vi "rsscope_core_global.vi"() -> ()   [LabVIEW 2018] (continued)
Options"="", "Flags"=0, "Help"="Defines for the selected field, how an index check is executed."}, {"Level"=5, "Class Only"=FALSE, "Identifier"="RSSCOPE_ATTR_USB_PD_SEARCH_INDEX_CONDITION", "Descriptive Name"="USB PD Search Index Condition", "Data Type"=0, "Command"="SEAR:TRIG:USBP:FRAM:FIEL{FieldNumber}:IOP", "Access"=2, "Range Table"="rsscope_rngUSB31Gen1IndexCondition", "Read Callback"="rsscope_FormatUSBPDPacketTypeInt32_ReadCallback.vi", "Write Callback"="rsscope_FormatUSBPDPacketTypeInt32_WriteCallback.vi", "Supported Models"="", "Instrument Options"="K63", "Flags"=0, "Help"="Sets the operator for the index in the selected field of the selected frame.\n\nAvailable Repeated Capabilities:\nFieldNumber: Field1, Field2, Field3, Field4, Field5, Field6, Field7, Field8, Field9, Field10, Field11, Field12, Field13, Field14, Field15, Field16, Field17, Field18, Field19, Field20\r\n\nRemote-control command(s):\nSEARch:TRIGger:USBPd:FRAMe:FIELd<m>:IOPerator"}, {"Level"=5, "Class Only"=FALSE, "Identifier"="RSSCOPE_ATTR_USB_PD_SEARCH_INDEX_MIN", "Descriptive Name"="USB PD Search Index Min", "Data Type"=0, "Command"="SEAR:TRIG:USBP:FRAM:FIEL{FieldNumber}:IMIN", "Access"=2, "Range Table"="", "Read Callback"="rsscope_FormatUSBPDPacketTypeInt32_ReadCallback.vi", "Write Callback"="rsscope_FormatUSBPDPacketTypeInt32_WriteCallback.vi", "Supported Models"="", "Instrument Options"="K63", "Flags"=0, "Help"="Specifies a data bit pattern, or sets the start value of a pattern range.\n\nValid Values:\nBinary pattern string consisting of 1; 0; or X (any bit).\n\nAvailable Repeated Capabilities:\nFieldNumber: Field1, Field2, Field3, Field4, Field5, Field6, Field7, Field8, Field9, Field10, Field11, Field12, Field13, Field14, Field15, Field16, Field17, Field18, Field19, Field20\r\n\nRemote-control command(s):\nSEARch:TRIGger:USBPd:FRAMe:FIELd<m>:IMIN"}, {"Level"=5, "Class Only"=FALSE, "Identifier"="RSSCOPE_ATTR_USB_PD_SEARCH_INDEX_MAX", "Descriptive Name"="USB PD Search Index Max", "Data Type"=0, "Command"="SEAR:TRIG:USBP:FRAM:FIEL{FieldNumber}:IMAX", "Access"=2, "Range Table"="", "Read Callback"="rsscope_FormatUSBPDPacketTypeInt32_ReadCallback.vi", "Write Callback"="rsscope_FormatUSBPDPacketTypeInt32_WriteCallback.vi", "Supported Models"="", "Instrument Options"="K63", "Flags"=0, "Help"="Sets the end value of a data type range for condition In Range or Out of Range. \n\nValid Values:\nBinary pattern string consisting of 1; 0; or X (any bit).\n\nAvailable Repeated Capabilities:\nFieldNumber: Field1, Field2, Field3, Field4, Field5, Field6, Field7, Field8, Field9, Field10, Field11, Field12, Field13, Field14, Field15, Field16, Field17, Field18, Field19, Field20\r\n\nRemote-control command(s):\nSEARch:TRIGger:USBPd:FRAMe:FIELd<m>:IMAX"}, {"Level"=4, "Class Only"=TRUE, "Identifier"="", "Descriptive Name"="Bit State", "Data Type"=0, "Command"="", "Access"=0, "Range Table"="", "Read Callback"="", "Write Callback"="", "Supported Models"="", "Instrument Options"="", "Flags"=0, "Help"="Defines the bit state to be checked for the selected field. Permitted bit states are 1, 0 or X (don&apos;t care)."}, {"Level"=5, "Class Only"=FALSE, "Identifier"="RSSCOPE_ATTR_USB_PD_SEARCH_BIT_STATE", "Descriptive Name"="USB PD Search Bit State", "Data Type"=0, "Command"="SEAR:TRIG:USBP:FRAM:FIEL{FieldNumber}:BIT", "Access"=2, "Range Table"="RsScope_rngBitState", "Read Callback"="rsscope_FormatUSBPDPacketTypeInt32_ReadCallback.vi", "Write Callback"="rsscope_FormatUSBPDPacketTypeInt32_WriteCallback.vi", "Supported Models"="", "Instrument Options"="K63", "Flags"=0, "Help"="Sets the bit state of a field that only consists of one bit.\n\nAvailable Repeated Capabilities:\nFieldNumber: Field1, Field2, Field3, Field4, Field5, Field6, Field7, Field8, Field9, Field10, Field11, Field12, Field13, Field14, Field15, Field16, Field17, Field18, Field19, Field20\r\n\nRemote-control command(s):\nSEARch:TRIGger:USBPd:FRAMe:FIELd<m>:BIT"}, {"Level"=4, "Class Only"=TRUE, "Identifier"="", "Descriptive Name"="Results", "Data Type"=0, "Command"="", "Access"=0, "Range Table"="", "Read Callback"="", "Write Callback"="", "Supported Models"="", "Instrument Options"="", "Flags"=0, "Help"="Returns the USB PD search results."}, {"Level"=5, "Class Only"=FALSE, "Identifier"="RSSCOPE_ATTR_SEARCH_USB_PD_FRAME_COUNT", "Descriptive Name"="Search USB PD Frame Count", "Data Type"=0, "Command"="SEAR:RES:USBP:FCO?", "Access"=0, "Range Table"="", "Read Callback"="rsscope_FormatSearchNameInt32_ReadCallback.vi", "Write Callback"="", "Supported Models"="", "Instrument Options"="K63", "Flags"=0, "Help"="Returns the number of frames in the acquisition.\n\nAvailable Repeated Capabilities:\nNone\n\nRemote-control command(s):\nSEARch:RESult:USBPd:FCOunt?"}, {"Level"=3, "Class Only"=TRUE, "Identifier"="", "Descriptive Name"="Custom Manchester NRZ", "Data Type"=0, "Command"="", "Access"=0, "Range Table"="", "Read Callback"="", "Write Callback"="", "Supported Models"="", "Instrument Options"="", "Flags"=0, "Help"="Configures Custom Manchester NRZ search"}, {"Level"=4, "Class Only"=TRUE, "Identifier"="", "Descriptive Name"="Results", "Data Type"=0, "Command"="", "Access"=0, "Range Table"="", "Read Callback"="", "Write Callback"="", "Supported Models"="", "Instrument Options"="", "Flags"=0, "Help"="Returns the search results."}, {"Level"=3, "Class Only"=TRUE, "Identifier"="", "Descriptive Name"="EbTb", "Data Type"=0, "Command"="", "Access"=0, "Range Table"="", "Read Callback"="", "Write Callback"="", "Supported Models"="", "Instrument Options"="", "Flags"=0, "Help"="The 8b/10b (Option R&S RTO-K52) coding scheme is used for high-speed serial data transmission, used by different standards, like fibre channel, PCIe, DVI and USB 3.0. Also the MIPI UniPro M-PHY interface in smartphones as well as display interfaces such as HDMI use 8b/10b encoding, as do base stations based on the Common Public Radio Interface (CPRI)."}, {"Level"=4, "Class Only"=FALSE, "Identifier"="RSSCOPE_ATTR_SEARCH_EBTB_TYPE", "Descriptive Name"="Search EbTb Type", "Data Type"=0, "Command"="SEAR:TRIG:EBTB:TYPE", "Access"=2, "Range Table"="RsScope_rngEbTbTriggerType", "Read Callback"="rsscope_FormatSearchNameInt32_ReadCallback.vi", "Write Callback"="rsscope_FormatSearchNameInt32_WriteCallback.vi", "Supported Models"="", "Instrument Options"="K52", "Flags"=0, "Help"="Selects the type of condition to be searched for. You can search for a certain symbol or enable a specific error condition.\n\nAvailable Repeated Capabilities:\nNone\n\nRemote-control command(s):\nSEARch:TRIGger:EBTB:TYPE"}, {"Level"=4, "Class Only"=FALSE, "Identifier"="RSSCOPE_ATTR_SEARCH_EBTB_DISPARITY_ERROR", "Descriptive Name"="Search EbTb Disparity Error", "Data Type"=3, "Command"="SEAR:TRIG:EBTB:DISP", "Access"=2, "Range Table"="", "Read Callback"="rsscope_FormatSearchNameBoolean_ReadCallback.vi", "Write Callback"="rsscope_FormatSearchNameBoolean_WriteCallback.vi", "Supported Models"="", "Instrument Options"="K52", "Flags"=0, "Help"="Searches for disparity errors.\n\nAvailable Repeated Capabilities:\nNone\n\nRemote-control command(s):\nSEARch:TRIGger:EBTB:DISParityerr"}, {"Level"=4, "Class Only"=FALSE, "Identifier"="RSSCOPE_ATTR_SEARCH_EBTB_GLITCHING_ERROR", "Descriptive Name"="Search EbTb Glitching Error", "Data Type"=3, "Command"="SEAR:TRIG:EBTB:GLIT", "Access"=2, "Range Table"="", "Read Callback"="rsscope_FormatSearchNameBoolean_ReadCallback.vi", "Write Callback"="rsscope_FormatSearchNameBoolean_WriteCallback.vi", "Supported Models"="", "Instrument Options"="K52", "Flags"=0, "Help"="Searches for glitching errors.\n\nAvailable Repeated Capabilities:\nNone\n\nRemote-control command(s):\nSEARch:TRIGger:EBTB:GLITcherror"}, {"Level"=4, "Class Only"=FALSE, "Identifier"="RSSCOPE_ATTR_SEARCH_EBTB_UNKNOWN_SYMBOL_ERROR", "Descriptive Name"="Search EbTb Unknown Symbol Error", "Data Type"=3, "Command"="SEAR:TRIG:EBTB:UNK", "Access"=2, "Range Table"="", "Read Callback"="rsscope_FormatSearchNameBoolean_ReadCallback.vi", "Write Callback"="rsscope_FormatSearchNameBoolean_WriteCallback.vi", "Supported Models"="", "Instrument Options"="K52", "Flags"=0, "Help"="Defines, whether a search for any unknown symbol error shall be activated or not.\n\nAvailable Repeated Capabilities:\nNone\n\nRemote-control command(s):\nSEARch:TRIGger:EBTB:UNK"}, {"Level"=4, "Class Only"=FALSE, "Identifier"="RSSCOPE_ATTR_SEARCH_EBTB_SEARCH_TYPE", "Descriptive Name"="Search EbTb Search Type", "Data Type"=0, "Command"="SEAR:TRIG:EBTB:STYP", "Access"=2, "Range Table"="RsScope_rngEbTbSearchType", "Read Callback"="rsscope_FormatSearchNameInt32_ReadCallback.vi", "Write Callback"="rsscope_FormatSearchNameInt32_WriteCallback.vi", "Supported Models"="", "Instrument Options"="K52", "Flags"=0, "Help"="Selects the search type.\n\nAvailable Repeated Capabilities:\nNone\n\nRemote-control command(s):\nSEARch:TRIGger:EBTB:STYPe"}, {"Level"=4, "Class Only"=FALSE, "Identifier"="RSSCOPE_ATTR_SEARCH_EBTB_SYMBOL_TYPE", "Descriptive Name"="Search EbTb Symbol Type", "Data Type"=0, "Command"="SEAR:TRIG:EBTB:SSTY", "Access"=2, "Range Table"="RsScope_rngEbTbSymbolType", "Read Callback"="rsscope_FormatSearchNameInt32_ReadCallback.vi", "Write Callback"="rsscope_FormatSearchNameInt32_WriteCallback.vi", "Supported Models"="", "Instrument Options"="K52", "Flags"=0, "Help"="Selects the symbol type to be searched for. You can select a single symbol or an expression (defined series of symbols).\n\nAvailable Repeated Capabilities:\nNone\n\nRemote-control command(s):\nSEARch:TRIGger:EBTB:SSTYpe"}, {"Level"=4, "Class Only"=FALSE, "Identifier"="RSSCOPE_ATTR_SEARCH_EBTB_SYMBOL_FORMAT", "Descriptive Name"="Search EbTb Symbol Format", "Data Type"=0, "Command"="SEAR:TRIG:EBTB:SYMF", "Access"=2, "Range Table"="RsScope_rngEbTbFormat", "Read Callback"="rsscope_FormatSearchNameInt32_ReadCallback.vi", "Write Callback"="rsscope_FormatSearchNameInt32_WriteCallback.vi", "Supported Models"="", "Instrument Options"="K52", "Flags"=0, "Help"="Selects the format of the symbol to be searched for, if &apos;Symbol Type&apos; > &apos;Symbol&apos;.\n\nAvailable Repeated Capabilities:\nNone\n\nRemote-control command(s):\nSEARch:TRIGger:EBTB:SYMFormat"}, {"Level"=4, "Class Only"=FALSE, "Identifier"="RSSCOPE_ATTR_SEARCH_EBTB_KD_CODE_SYMBOL", "Descriptive Name"="Search EbTb KD Code Symbol", "Data Type"=0, "Command"="SEAR:TRIG:EBTB:SYMT", "Access"=2, "Range Table"="RsScope_rngEbTbKDCode", "Read Callback"="rsscope_FormatSearchNameInt32_ReadCallback.vi", "Write Callback"="rsscope_FormatSearchNameInt32_WriteCallback.vi", "Supported Models"="", "Instrument Options"="K52", "Flags"=0, "Help"="Selects the data character (Dx.y) or control character to be searched for. You can specify the value of the data character to be searched for with &apos;Dx Value&apos; and &apos;Dy Value&apos;.\n\nAvailable Repeated Capabilities:\nNone\n\nRemote-control command(s):\nSEARch:TRIGger:EBTB:SYMType"}, {"Level"=4, "Class Only"=FALSE, "Identifier"="RSSCOPE_ATTR_SEARCH_EBTB_DX", "Descriptive Name"="Search EbTb Dx", "Data Type"=0, "Command"="SEAR:TRIG:EBTB:DX", "Access"=2, "Range Table"="RsScope_rngEbTbDx", "Read Callback"="rsscope_FormatSearchNameInt32_ReadCallback.vi", "Write Callback"="rsscope_FormatSearchNameInt32_WriteCallback.vi", "Supported Models"="", "Instrument Options"="K52", "Flags"=0, "Help"="Sets the x value of the data character Dx.y to be searched for, if &apos;K/D Codes Symbol&apos; > &apos;Dx.y&apos;.\n\nAvailable Repeated Capabilities:\nNone\n\nRemote-control command(s):\nSEARch:TRIGger:EBTB:DX"}, {"Level"=4, "Class Only"=FALSE, "Identifier"="RSSCOPE_ATTR_SEARCH_EBTB_DY", "Descriptive Name"="Search EbTb Dy", "Data Type"=0, "Command"="SEAR:TRIG:EBTB:DY", "Access"=2, "Range Table"="RsScope_rngEbTbDy", "Read Callback"="rsscope_FormatSearchNameInt32_ReadCallback.vi", "Write Callback"="rsscope_FormatSearchNameInt32_WriteCallback.vi", "Supported Models"="", "Instrument Options"="K52", "Flags"=0, "Help"="Sets the y value of the data character Dx.y to be searched for, if &apos;K/D Codes Symbol&apos; > &apos;Dx.y&apos;.\n\nAvailable Repeated Capabilities:\nNone\n\nRemote-control command(s):\nSEARch:TRIGger:EBTB:DY"}, {"Level"=4, "Class Only"=FALSE, "Identifier"="RSSCOPE_ATTR_SEARCH_EBTB_EIGHT_BIT_PATTERN", "Descriptive Name"="Search EBTB Eight Bit Pattern", "Data Type"=2, "Command"="SEAR:TRIG:EBTB:EBPA", "Access"=2, "Range Table"="", "Read Callback"="rsscope_FormatSearchNameString_ReadCallback.vi", "Write Callback"="rsscope_FormatSearchNameString_WriteCallback.vi", "Supported Models"="", "Instrument Options"="K52", "Flags"=0, "Help"="Sets the 8-bit pattern to be searched for, if &apos;Format&apos; > &apos;8-bit&apos;.\n \nNote(s):\n(1) Valid values 1; 0; or X (any bit), use of X is restricted to the conditions &apos;Equal&apos; and &apos;Not equal&apos;.\n\nAvailable Repeated Capabilities:\nNone\n\nRemote-control command(s):\nSEARch:TRIGger:EBTB:EBPA"}, {"Level"=4, "Class Only"=FALSE, "Identifier"="RSSCOPE_ATTR_SEARCH_EBTB_TEN_BIT_PATTERN", "Descriptive Name"="Search EBTB Ten Bit Pattern", "Data Type"=2, "Command"="SEAR:TRIG:EBTB:TBPA", "Access"=2, "Range Table"="", "Read Callback"="rsscope_FormatSearchNameString_ReadCallback.vi", "Write Callback"="rsscope_FormatSearchNameString_WriteCallback.vi", "Supported Models"="", "Instrument Options"="K52", "Flags"=0, "Help"="Sets the 10-bit pattern to be searched for, if &apos;Format&apos; > &apos;10-bit&apos;.\n \nNote(s):\n(1) Valid values 1; 0; or X (any bit), use of X is restricted to the conditions &apos;Equal&apos; and &apos;Not equal&apos;.\n\nAvailable Repeated Capabilities:\nNone\n\nRemote-control command(s):\nSEARch:TRIGger:EBTB:TBPA"}, {"Level"=4, "Class Only"=FALSE, "Identifier"="RSSCOPE_ATTR_SEARCH_EBTB_EXPRESSION", "Descriptive Name"="Search EBTB Expression", "Data Type"=2, "Command"="SEAR:TRIG:EBTB:SYME", "Access"=2, "Range Table"="", "Read Callback"="rsscope_FormatSearchNameString_ReadCallback.vi", "Write Callback"="rsscope_FormatSearchNameString_WriteCallback.vi", "Supported Models"="", "Instrument Options"="K52", "Flags"=0, "Help"="Defines the expression to be searched for, if &apos;Symbol Type&apos; > &apos;Expression&apos;.\n\nAvailable Repeated Capabilities:\nNone\n\nRemote-control command(s):\nSEARch:TRIGger:EBTB:SYME"}, {"Level"=4, "Class Only"=TRUE, "Identifier"="", "Descriptive Name"="Results", "Data Type"=0, "Command"="", "Access"=0, "Range Table"="", "Read Callback"="", "Write Callback"="", "Supported Models"="", "Instrument Options"="", "Flags"=0, "Help"="Returns the search results."}, {"Level"=5, "Class Only"=FALSE, "Identifier"="RSSCOPE_ATTR_SEARCH_EBTB_SYMBOL_COUNT", "Descriptive Name"="Search EbTb Symbol Count", "Data Type"=0, "Command"="SEAR:RES:EBTB:SCO?", "Access"=0, "Range Table"="", "Read Callback"="rsscope_FormatSearchNameInt32_ReadCallback.vi", "Write Callback"="", "Supported Models"="", "Instrument Options"="K52", "Flags"=0, "Help"="Returns the symbol count for the selected serial bus, i.e. the number of symbols in the present acquisition.\n\nAvailable Repeated Capabilities:\nNone\n\nRemote-control command(s):\nSEARch:RESult:EBTB:SCOunt?"}, {"Level"=3, "Class Only"=TRUE, "Identifier"="", "Descriptive Name"="SENT", "Data Type"=0, "Command"="", "Access"=0, "Range Table"="", "Read Callback"="", "Write Callback"="", "Supported Models"="", "Instrument Options"="", "Flags"=0, "Help"="SENT (Single Ended Nibble Transmission, R&S RTO-K10 option) is a serial transmission interface protocol originally specified for the communication of sensors and control units in automotive electronics."}, {"Level"=4, "Class Only"=FALSE, "Identifier"="RSSCOPE_ATTR_SEARCH_SENT_CALIBRATION_ENABLED", "Descriptive Name"="Search SENT Calibration Enabled", "Data Type"=3, "Command"="SEAR:TRIG:SENT:CAL", "Access"=2, "Range Table"="", "Read Callback"="rsscope_FormatSearchNameBoolean_ReadCallback.vi", "Write Callback"="rsscope_FormatSearchNameBoolean_WriteCallback.vi", "Supported Models"="", "Instrument Options"="K10", "Flags"=0, "Help"="Enables the search for the Calibration/Synchronization pulse.\n\nAvailable Repeated Capabilities:\nNone\n\nRemote-control command(s):\nSEARch:TRIGger:SENT:CALibration"}, {"Level"=4, "Class Only"=TRUE, "Identifier"="", "Descriptive Name"="Transmission Sequence", "Data Type"=0, "Command"="", "Access"=0, "Range Table"="", "Read Callback"="", "Write Callback"="", "Supported Models"="", "Instrument Options"="", "Flags"=0, "Help"="Configures the trigger conditions for trigger type transmission sequence."}, {"Level"=5, "Class Only"=FALSE, "Identifier"="RSSCOPE_ATTR_SEARCH_SENT_TRANSMISSION_SEQUENCE_ENABLED", "Descriptive Name"="Search SENT Transmission Sequence Enabled", "Data Type"=3, "Command"="SEAR:TRIG:SENT:TRAN", "Access"=2, "Range Table"="", "Read Callback"="rsscope_FormatSearchNameBoolean_ReadCallback.vi", "Write Callback"="rsscope_FormatSearchNameBoolean_WriteCallback.vi", "Supported Models"="", "Instrument Options"="K10", "Flags"=0, "Help"="Enables the search for a transmission sequence.\n\nAvailable Repeated Capabilities:\nNone\n\nRemote-control command(s):\nSEARch:TRIGger:SENT:TRANsmission"}, {"Level"=5, "Class Only"=FALSE, "Identifier"="RSSCOPE_ATTR_SEARCH_SENT_TRANSMISSION_SEQUENCE_TYPE", "Descriptive Name"="Search SENT Transmission Sequence Type", "Data Type"=0, "Command"="SEAR:TRIG:SENT:TTYP", "Access"=2, "Range Table"="RsScope_rngSENTTriggerTSType", "Read Callback"="rsscope_FormatSearchNameInt32_ReadCallback.vi", "Write Callback"="rsscope_FormatSearchNameInt32_WriteCallback.vi", "Supported Models"="", "Instrument Options"="K10", "Flags"=0, "Help"="Selects the SENT transmission sequence to be searched for.\n\nAvailable Repeated Capabilities:\nNone\n\nRemote-control command(s):\nSEARch:TRIGger:SENT:TTYPe"}, {"Level"=5, "Class Only"=FALSE, "Identifier"="RSSCOPE_ATTR_SEARCH_SENT_TRANSMISSION_SEQUENCE_STATUS", "Descriptive Name"="Search SENT Transmission Sequence Status", "Data Type"=2, "Command"="SEAR:TRIG:SENT:STAT", "Access"=2, "Range Table"="", "Read Callback"="rsscope_FormatSearchNameString_ReadCallback.vi", "Write Callback"="rsscope_FormatSearchNameString_WriteCallback.vi", "Supported Models"="", "Instrument Options"="K10", "Flags"=0, "Help"="Sets the status nibble data, numeric or string pattern. The string parameter accepts the bit value X (don&apos;t care).\n\nAvailable Repeated Capabilities:\nNone\n\nRemote-control command(s):\nSEARch:TRIGger:SENT:STATus"}, {"Level"=5, "Class Only"=FALSE, "Identifier"="RSSCOPE_ATTR_SEARCH_SENT_TRANSMISSION_SEQUENCE_CONDITION", "Descriptive Name"="Search SENT Transmission Sequence Condition", "Data Type"=0, "Command"="SEAR:TRIG:SENT:TDCN", "Access"=2, "Range Table"="rsscope_rngProtocolTriggerCondition", "Read Callback"="rsscope_FormatSearchNameInt32_ReadCallback.vi", "Write Callback"="rsscope_FormatSearchNameInt32_WriteCallback.vi", "Supported Models"="", "Instrument Options"="K10", "Flags"=0, "Help"="Sets the operator to set a specific data pattern or a data pattern range.\n\nAvailable Repeated Capabilities:\nNone\n\nRemote-control command(s):\nSEARch:TRIGger:SENT:TDCN"}, {"Level"=5, "Class Only"=FALSE, "Identifier"="RSSCOPE_ATTR_SEARCH_SENT_TRANSMISSION_SEQUENCE_DATA_MIN", "Descriptive Name"="Search SENT Transmission Sequence Data Min", "Data Type"=2, "Command"="SEAR:TRIG:SENT:TDMN", "Access"=2, "Range Table"="", "Read Callback"="rsscope_FormatSearchNameString_ReadCallback.vi", "Write Callback"="rsscope_FormatSearchNameString_WriteCallback.vi", "Supported Models"="", "Instrument Options"="K10", "Flags"=0, "Help"="Specifies a data pattern, or sets the start value of a data pattern range. The string parameter accepts the bit value X (don&apos;t care).\n\nAvailable Repeated Capabilities:\nNone\n\nRemote-control command(s):\nSEARch:TRIGger:SENT:TDMN"}, {"Level"=5, "Class Only"=FALSE, "Identifier"="RSSCOPE_ATTR_SEARCH_SENT_TRANSMISSION_SEQUENCE_DATA_MAX", "Descriptive Name"="Search SENT Transmission Sequence Data Max", "Data Type"=2, "Command"="SEAR:TRIG:SENT:TDMX", "Access"=2, "Range Table"="", "Read Callback"="rsscope_FormatSearchNameString_ReadCallback.vi", "Write Callback"="rsscope_FormatSearchNameString_WriteCallback.vi", "Supported Models"="", "Instrument Options"="K10", "Flags"=0, "Help"="Sets the end value of an identifier range for condition In Range or Out of Range. The string parameter accepts the bit value X (don&apos;t care).\n\nAvailable Repeated Capabilities:\nNone\n\nRemote-control command(s):\nSEARch:TRIGger:SENT:TDMX"}, {"Level"=4, "Class Only"=TRUE, "Identifier"="", "Descriptive Name"="Serial Message", "Data Type"=0, "Command"="", "Access"=0, "Range Table"="", "Read Callback"="", "Write Callback"="", "Supported Models"="", "Instrument Options"="", "Flags"=0, "Help"="Configures the trigger conditions for a serial message."}, {"Level"=5, "Class Only"=FALSE, "Identifier"="RSSCOPE_ATTR_SEARCH_SENT_SERIAL_MESSAGE_ENABLED", "Descriptive Name"="Search SENT Serial Message Enabled", "Data Type"=3, "Command"="SEAR:TRIG:SENT:SMSG", "Access"=2, "Range Table"="", "Read Callback"="rsscope_FormatSearchNameBoolean_ReadCallback.vi", "Write Callback"="rsscope_FormatSearchNameBoolean_WriteCallback.vi", "Supported Models"="", "Instrument Options"="K10", "Flags"=0, "Help"="Enables the search in a serial message.\n\nAvailable Repeated Capabilities:\nNone\n\nRemote-control command(s):\nSEARch:TRIGger:SENT:SMSG"}, {"Level"=5, "Class Only"=FALSE, "Identifier"="RSSCOPE_ATTR_SEARCH_SENT_SERIAL_MESSAGE_TYPE", "Descriptive Name"="Search SENT Serial Message Type", "Data Type"=0, "Command"="SEAR:TRIG:SENT:STYP", "Access"=2, "Range Table"="RsScope_rngSENTTriggerSMType", "Read Callback"="rsscope_FormatSearchNameInt32_ReadCallback.vi", "Write Callback"="rsscope_FormatSearchNameInt32_WriteCallback.vi", "Supported Models"="", "Instrument Options"="K10", "Flags"=0, "Help"="Selects the serial message sequence to be searched for.\n\nAvailable Repeated Capabilities:\nNone\n\nRemote-control command(s):\nSEARch:TRIGger:SENT:STYPe"}, {"Level"=5, "Class Only"=FALSE, "Identifier"="RSSCOPE_ATTR_SEARCH_SENT_SERIAL_MESSAGE_ID_TYPE", "Descriptive Name"="Search SENT Serial Message ID Type", "Data Type"=0, "Command"="SEAR:TRIG:SENT:SIDT", "Access"=2, "Range Table"="RsScope_rngSENTIDType", "Read Callback"="rsscope_FormatSearchNameInt32_ReadCallback.vi", "Write Callback"="rsscope_FormatSearchNameInt32_WriteCallback.vi", "Supported Models"="", "Instrument Options"="K10", "Flags"=0, "Help"="Sets the message ID format (4 bit or 8 bit) of the enhanced serial message.\n\nAvailable Repeated Capabilities:\nNone\n\nRemote-control command(s):\nSEARch:TRIGger:SENT:SIDType"}, {"Level"=5, "Class Only"=FALSE, "Identifier"="RSSCOPE_ATTR_SEARCH_SENT_SERIAL_MESSAGE_ID_CONDITION", "Descriptive Name"="Search SENT Serial Message ID Condition", "Data Type"=0, "Command"="SEAR:TRIG:SENT:SICN", "Access"=2, "Range Table"="rsscope_rngProtocolTriggerCondition", "Read Callback"="rsscope_FormatSearchNameInt32_ReadCallback.vi", "Write Callback"="rsscope_FormatSearchNameInt32_WriteCallback.vi", "Supported Models"="", "Instrument Options"="K10", "Flags"=0, "Help"="Sets the operator to set a specific data pattern or a data pattern range.\n\nAvailable Repeated Capabilities:\nNone\n\nRemote-control command(s):\nSEARch:TRIGger:SENT:SICN"}, {"Level"=5, "Class Only"=FALSE, "Identifier"="RSSCOPE_ATTR_SEARCH_SENT_SERIAL_MESSAGE_ID_MIN", "Descriptive Name"="Search SENT Serial Message ID Min", "Data Type"=2, "Command"="SEAR:TRIG:SENT:SIMN", "Access"=2, "Range Table"="", "Read Callback"="rsscope_FormatSearchNameString_ReadCallback.vi", "Write Callback"="rsscope_FormatSearchNameString_WriteCallback.vi", "Supported Models"="", "Instrument Options"="K10", "Flags"=0, "Help"="Specifies a message identifier pattern, or sets the start value of an identifier range. The string parameter accepts the bit value X (don&apos;t care).\n\nAvailable Repeated Capabilities:\nNone\n\nRemote-control command(s):\nSEARch:TRIGger:SENT:SIMN"}, {"Level"=5, "Class Only"=FALSE, "Identifier"="RSSCOPE_ATTR_SEARCH_SENT_SERIAL_MESSAGE_ID_MAX", "Descriptive Name"="Search SENT Serial Message ID Max", "Data Type"=2, "Command"="SEAR:TRIG:SENT:SIMX", "Access"=2, "Range Table"="", "Read Callback"="rsscope_FormatSearchNameString_ReadCallback.vi", "Write Callback"="rsscope_FormatSearchNameString_WriteCallback.vi", "Supported Models"="", "Instrument Options"="K10", "Flags"=0, "Help"="Sets the end value of an identifier range for condition In Range or Out of Range. The string parameter accepts the bit value X (don&apos;t care).\n\nAvailable Repeated Capabilities:\nNone\n\nRemote-control command(s):\nSEARch:TRIGger:SENT:SIMX"}, {"Level"=5, "Class Only"=FALSE, "Identifier"="RSSCOPE_ATTR_SEARCH_SENT_SERIAL_MESSAGE_DATA_CONDITION", "Descriptive Name"="Search SENT Serial Message Data Condition", "Data Type"=0, "Command"="SEAR:TRIG:SENT:SDCN", "Access"=2, "Range Table"="rsscope_rngProtocolTriggerCondition", "Read Callback"="rsscope_FormatSearchNameInt32_ReadCallback.vi", "Write Callback"="rsscope_FormatSearchNameInt32_WriteCallback.vi", "Supported Models"="", "Instrument Options"="K10", "Flags"=0, "Help"="Sets the operator to define a specific data pattern or a data pattern range.\n\nAvailable Repeated Capabilities:\nNone\n\nRemote-control command(s):\nSEARch:TRIGger:SENT:SDCN"}, {"Level"=5, "Class Only"=FALSE, "Identifier"="RSSCOPE_ATTR_SEARCH_SENT_SERIAL_MESSAGE_DATA_MIN", "Descriptive Name"="Search SENT Serial Message Data Min", "Data Type"=2, "Command"="SEAR:TRIG:SENT:SDMN", "Access"=2, "Range Table"="", "Read Callback"="rsscope_FormatSearchNameString_ReadCallback.vi", "Write Callback"="rsscope_FormatSearchNameString_WriteCallback.vi", "Supported Models"="", "Instrument Options"="K10", "Flags"=0, "Help"="Specifies a data pattern, or sets the start value of a data pattern range. The string parameter accepts the bit value X (don&apos;t care).\n\nAvailable Repeated Capabilities:\nNone\n\nRemote-control command(s):\nSEARch:TRIGger:SENT:SDMN"}, {"Level"=5, "Class Only"=FALSE, "Identifier"="RSSCOPE_ATTR_SEARCH_SENT_SERIAL_MESSAGE_DATA_MAX", "Descriptive Name"="Search SENT Serial Message Data Max", "Data Type"=2, "Command"="SEAR:TRIG:SENT:SDMX", "Access"=2, "Range Table"="", "Read Callback"="rsscope_FormatSearchNameString_ReadCallback.vi", "Write Callback"="rsscope_FormatSearchNameString_WriteCallback.vi", "Supported Models"="", "Instrument Options"="K10", "Flags"=0, "Help"="Sets the end value of an identifier range for condition In Range or Out of Range. The string parameter accepts the bit value X (don&apos;t care).\n\nAvailable Repeated Capabilities:\nNone\n\nRemote-control command(s):\nSEARch:TRIGger:SENT:SDMX"}, {"Level"=4, "Class Only"=TRUE, "Identifier"="", "Descriptive Name"="Error Conditions", "Data Type"=0, "Command"="", "Access"=0, "Range Table"="", "Read Callback"="", "Write Callback"="", "Supported Models"="", "Instrument Options"="", "Flags"=0, "Help"="This class configures conditions for Error trigger."}, {"Level"=5, "Class Only"=FALSE, "Identifier"="RSSCOPE_ATTR_SEARCH_SENT_ERROR_ENABLED", "Descriptive Name"="Search SENT Error Enabled", "Data Type"=3, "Command"="SEAR:TRIG:SENT:ERR", "Access"=2, "Range Table"="", "Read Callback"="rsscope_FormatSearchNameBoolean_ReadCallback.vi", "Write Callback"="rsscope_FormatSearchNameBoolean_WriteCallback.vi", "Supported Models"="", "Instrument Options"="K10", "Flags"=0, "Help"="Enables the search for a specified error.\n\nAvailable Repeated Capabilities:\nNone\n\nRemote-control command(s):\nSEARch:TRIGger:SENT:ERRor"}, {"Level"=5, "Class Only"=FALSE, "Identifier"="RSSCOPE_ATTR_SEARCH_SENT_FORM_ERROR", "Descriptive Name"="Search SENT Form Error", "Data Type"=3, "Command"="SEAR:TRIG:SENT:FORM", "Access"=2, "Range Table"="", "Read Callback"="rsscope_FormatSearchNameBoolean_ReadCallback.vi", "Write Callback"="rsscope_FormatSearchNameBoolean_WriteCallback.vi", "Supported Models"="", "Instrument Options"="K10", "Flags"=0, "Help"="Enables the search for format errors in serial messages.\n\nAvailable Repeated Capabilities:\nNone\n\nRemote-control command(s):\nSEARch:TRIGger:SENT:FORMerror"}, {"Level"=5, "Class Only"=FALSE, "Identifier"="RSSCOPE_ATTR_SEARCH_SENT_CALIBRATION_PULSE_ERROR", "Descriptive Name"="Search SENT Calibration Pulse Error", "Data Type"=3, "Command"="SEAR:TRIG:SENT:PULS", "Access"=2, "Range Table"="", "Read Callback"="rsscope_FormatSearchNameBoolean_ReadCallback.vi", "Write Callback"="rsscope_FormatSearchNameBoolean_WriteCallback.vi", "Supported Models"="", "Instrument Options"="K10", "Flags"=0, "Help"="Enables the search for pulse errors.\n\nAvailable Repeated Capabilities:\nNone\n\nRemote-control command(s):\nSEARch:TRIGger:SENT:PULSeerror"}, {"Level"=5, "Class Only"=FALSE, "Identifier"="RSSCOPE_ATTR_SEARCH_SENT_PULSE_PERIOD_ERROR", "Descriptive Name"="Search SENT Pulse Period Error", "Data Type"=3, "Command"="SEAR:TRIG:SENT:PPER", "Access"=2, "Range Table"="", "Read Callback"="rsscope_FormatSearchNameBoolean_ReadCallback.vi", "Write Callback"="rsscope_FormatSearchNameBoolean_WriteCallback.vi", "Supported Models"="", "Instrument Options"="K10", "Flags"=0, "Help"="Enables the search for pulse period errors.\n\nAvailable Repeated Capabilities:\nNone\n\nRemote-control command(s):\nSEARch:TRIGger:SENT:PPERioderror"}, {"Level"=5, "Class Only"=FALSE, "Identifier"="RSSCOPE_ATTR_SEARCH_SENT_CRC_ERROR", "Descriptive Name"="Search SENT CRC Error", "Data Type"=3, "Command"="SEAR:TRIG:SENT:CRC", "Access"=2, "Range Table"="", "Read Callback"="rsscope_FormatSearchNameBoolean_ReadCallback.vi", "Write Callback"="rsscope_FormatSearchNameBoolean_WriteCallback.vi", "Supported Models"="", "Instrument Options"="K10", "Flags"=0, "Help"="Enables the search for errors in the Cyclic Redundancy Check.\n\nAvailable Repeated Capabilities:\nNone\n\nRemote-control command(s):\nSEARch:TRIGger:SENT:CRCerror"}, {"Level"=5, "Class Only"=FALSE, "Identifier"="RSSCOPE_ATTR_SEARCH_SENT_IRREGULAR_FRAME_LENGTH_ERROR", "Descriptive Name"="Search SENT Irregular Frame Length Error", "Data Type"=3, "Command"="SEAR:TRIG:SENT:IRFL", "Access"=2, "Range Table"="", "Read Callback"="rsscope_FormatSearchNameBoolean_ReadCallback.vi", "Write Callback"="rsscope_FormatSearchNameBoolean_WriteCallback.vi", "Supported Models"="", "Instrument Options"="K10", "Flags"=0, "Help"="Enables the search for irregular frame length errors.\n\nAvailable Repeated Capabilities:\nNone\n\nRemote-control command(s):\nSEARch:TRIGger:SENT:IRFLength"}, {"Level"=4, "Class Only"=TRUE, "Identifier"="", "Descriptive Name"="Results", "Data Type"=0, "Command"="", "Access"=0, "Range Table"="", "Read Callback"="", "Write Callback"="", "Supported Models"="", "Instrument Options"="", "Flags"=0, "Help"="Returns the search results."}, {"Level"=5, "Class Only"=FALSE, "Identifier"="RSSCOPE_ATTR_SEARCH_SENT_FRAME_COUNT", "Descriptive Name"="Search SENT Frame Count", "Data Type"=0, "Command"="SEAR:RES:SENT:FCO?", "Access"=0, "Range Table"="", "Read Callback"="rsscope_FormatSearchNameInt32_ReadCallback.vi", "Write Callback"="", "Supported Models"="", "Instrument Options"="K10", "Flags"=0, "Help"="Returns the number of decoded frames of the acquisition.\n\nAvailable Repeated Capabilities:\nNone\n\nRemote-control command(s):\nSEARch:RESult:SENT:FCOunt?"}, {"Level"=3, "Class Only"=TRUE, "Identifier"="", "Descriptive Name"="D-PHY", "Data Type"=0, "Command"="", "Access"=0, "Range Table"="", "Read Callback"="", "Write Callback"="", "Supported Models"="", "Instrument Options"="", "Flags"=0, "Help"="In this class all search settings can be configured."}, {"Level"=4, "Class Only"=FALSE, "Identifier"="RSSCOPE_ATTR_DPHY_SEARCH_TYPE", "Descriptive Name"="DPHY Search Type", "Data Type"=0, "Command"="SEAR:TRIG:DPHY:TYPE", "Access"=2, "Range Table"="RsScope_rngDPHYTriggerType", "Read Callback"="rsscope_FormatSearchNameInt32_ReadCallback.vi", "Write Callback"="rsscope_FormatSearchNameInt32_WriteCallback.vi", "Supported Models"="", "Instrument Options"="K42", "Flags"=0, "Help"="Sets the type of frame to be searched for.\n\nAvailable Repeated Capabilities:\nNone\n\nRemote-control command(s):\nSEARch:TRIGger:DPHY:TYPE"}, {"Level"=4, "Class Only"=FALSE, "Identifier"="RSSCOPE_ATTR_DPHY_SEARCH_VIRTUAL_CHANNEL", "Descriptive Name"="DPHY Search Virtual Channel", "Data Type"=2, "Command"="SEAR:TRIG:DPHY:HSVC", "Access"=2, "Range Table"="", "Read Callback"="rsscope_FormatSearchNameString_ReadCallback.vi", "Write Callback"="rsscope_FormatSearchNameString_WriteCallback.vi", "Supported Models"="", "Instrument Options"="K42", "Flags"=0, "Help"="Sets the virtual channel to be searched for.\n\nAvailable Repeated Capabilities:\nNone\n\nRemote-control command(s):\nSEARch:TRIGger:DPHY:HSVC"}, {"Level"=4, "Class Only"=TRUE, "Identifier"="", "Descriptive Name"="Data Type", "Data Type"=0, "Command"="", "Access"=0, "Range Table"="", "Read Callback"="", "Write Callback"="", "Supported Models"="", "Instrument Options"="", "Flags"=0, "Help"="Sets the specified data type to be searched for. The data type setup consists of the condition and one or two data patterns."}, {"Level"=5, "Class Only"=FALSE, "Identifier"="RSSCOPE_ATTR_DPHY_SEARCH_DATA_TYPE_CONDITION", "Descriptive Name"="DPHY Search Data Type Condition", "Data Type"=0, "Command"="SEAR:TRIG:DPHY:DTYP:COND", "Access"=2, "Range Table"="rsscope_rngProtocolTriggerCondition", "Read Callback"="rsscope_FormatSearchNameInt32_ReadCallback.vi", "Write Callback"="rsscope_FormatSearchNameInt32_WriteCallback.vi", "Supported Models"="", "Instrument Options"="K42", "Flags"=0, "Help"="Set the condition for the data type. You can define an exact value or a value range.\n\nAvailable Repeated Capabilities:\nNone\n\nRemote-control command(s):\nSEARch:TRIGger:DPHY:DTYPe:CONDition"}, {"Level"=5, "Class Only"=FALSE, "Identifier"="RSSCOPE_ATTR_DPHY_SEARCH_DATA_TYPE_MIN", "Descriptive Name"="DPHY Search Data Type Min", "Data Type"=2, "Command"="SEAR:TRIG:DPHY:DTYP:MIN", "Access"=2, "Range Table"="", "Read Callback"="", "Write Callback"="", "Supported Models"="", "Instrument Options"="K42", "Flags"=0, "Help"="Specifies a data type pattern, or sets the start value of a pattern range.\n\nValid Values:\nBinary pattern string consisting of 1; 0; or X (any bit).\n\nAvailable Repeated Capabilities:\nNone\n\nRemote-control command(s):\nSEARch:TRIGger:DPHY:DTYPe:MIN"}, {"Level"=5, "Class Only"=FALSE, "Identifier"="RSSCOPE_ATTR_DPHY_SEARCH_DATA_TYPE_MAX", "Descriptive Name"="DPHY Search Data Type Max", "Data Type"=2, "Command"="SEAR:TRIG:DPHY:DTYP:MAX", "Access"=2, "Range Table"="", "Read Callback"="rsscope_FormatSearchNameString_ReadCallback.vi", "Write Callback"="rsscope_FormatSearchNameString_WriteCallback.vi", "Supported Models"="", "Instrument Options"="K42", "Flags"=0, "Help"="Sets the end value of a data type range for condition In Range or Out of Range. \n\nValid Values:\nBinary pattern string consisting of 1; 0; or X (any bit).\n\nAvailable Repeated Capabilities:\nNone\n\nRemote-control command(s):\nSEARch:TRIGger:DPHY:DTYPe:MAX"}, {"Level"=4, "Class Only"=TRUE, "Identifier"="", "Descriptive Name"="Word Count", "Data Type"=0, "Command"="", "Access"=0, "Range Table"="", "Read Callback"="", "Write Callback"="", "Supported Models"="", "Instrument Options"="", "Flags"=0, "Help"="Sets the specified data type to be searched for. The word count setup consists of the condition and one or two data patterns."}, {"Level"=5, "Class Only"=FALSE, "Identifier"="RSSCOPE_ATTR_DPHY_SEARCH_WORD_COUNT_CONDITION", "Descriptive Name"="DPHY Search Word Count Condition", "Data Type"=0, "Command"="SEAR:TRIG:DPHY:WCO:COND", "Access"=2, "Range Table"="rsscope_rngProtocolTriggerCondition", "Read Callback"="rsscope_FormatSearchNameInt32_ReadCallback.vi", "Write Callback"="rsscope_FormatSearchNameInt32_WriteCallback.vi", "Supported Models"="", "Instrument Options"="K42", "Flags"=0, "Help"="Set the condition for the word count. You can define an exact value or a value range.\n\nAvailable Repeated Capabilities:\nNone\n\nRemote-control command(s):\nSEARch:TRIGger:DPHY:WCOunt:CONDition"}, {"Level"=5, "Class Only"=FALSE, "Identifier"="RSSCOPE_ATTR_DPHY_SEARCH_WORD_COUNT_MIN", "Descriptive Name"="DPHY Search Word Count Min", "Data Type"=2, "Command"="SEAR:TRIG:DPHY:WCO:MIN", "Access"=2, "Range Table"="", "Read Callback"="rsscope_FormatSearchNameString_ReadCallback.vi", "Write Callback"="rsscope_FormatSearchNameString_WriteCallback.vi", "Supported Models"="", "Instrument Options"="K42", "Flags"=0, "Help"="Specifies a word bit pattern, or sets the start value of a pattern range.\n\nValid Values:\nBinary pattern string consisting of 1; 0; or X (any bit).\n\nAvailable Repeated Capabilities:\nNone\n\nRemote-control command(s):\nSEARch:TRIGger:DPHY:WCOunt:MIN"}, {"Level"=5, "Class Only"=FALSE, "Identifier"="RSSCOPE_ATTR_DPHY_SEARCH_WORD_COUNT_MAX", "Descriptive Name"="DPHY Search Word Count Max", "Data Type"=2, "Command"="SEAR:TRIG:DPHY:WCO:MAX", "Access"=2, "Range Table"="", "Read Callback"="rsscope_FormatSearchNameString_ReadCallback.vi", "Write Callback"="rsscope_FormatSearchNameString_WriteCallback.vi", "Supported Models"="", "Instrument Options"="K42", "Flags"=0, "Help"="Sets the end value of a data type range for condition In Range or Out of Range. \n\nValid Values:\nBinary pattern string consisting of 1; 0; or X (any bit).\n\nAvailable Repeated Capabilities:\nNone\n\nRemote-control command(s):\nSEARch:TRIGger:DPHY:WCOunt:MAX"}, {"Level"=4, "Class Only"=TRUE, "Identifier"="", "Descriptive Name"="Data", "Data Type"=0, "Command"="", "Access"=0, "Range Table"="", "Read Callback"="", "Write Callback"="", "Supported Models"="", "Instrument Options"="", "Flags"=0, "Help"="Set the specified data value to be searched for.The data value setup consists of the\ncondition and one or two data value patterns."}, {"Level"=5, "Class Only"=FALSE, "Identifier"="RSSCOPE_ATTR_DPHY_SEARCH_HIGH_SPEED_DATA_CONDITION", "Descriptive Name"="DPHY Search High Speed Data Condition", "Data Type"=0, "Command"="SEAR:TRIG:DPHY:DATA:COND", "Access"=2, "Range Table"="rsscope_rngProtocolTriggerCondition", "Read Callback"="rsscope_FormatSearchNameInt32_ReadCallback.vi", "Write Callback"="rsscope_FormatSearchNameInt32_WriteCallback.vi", "Supported Models"="", "Instrument Options"="K42", "Flags"=0, "Help"="Set the condition for the data value. You can define an exact value or a value range.\n\nAvailable Repeated Capabilities:\nNone\n\nRemote-control command(s):\nSEARch:TRIGger:DPHY:DATA:CONDition"}, {"Level"=5, "Class Only"=FALSE, "Identifier"="RSSCOPE_ATTR_DPHY_SEARCH_HIGH_SPEED_DATA_MIN", "Descriptive Name"="DPHY Search High Speed Data Min", "Data Type"=2, "Command"="SEAR:TRIG:DPHY:DATA:MIN", "Access"=2, "Range Table"="", "Read Callback"="rsscope_FormatSearchNameString_ReadCallback.vi", "Write Callback"="rsscope_FormatSearchNameString_WriteCallback.vi", "Supported Models"="", "Instrument Options"="K42", "Flags"=0, "Help"="Specifies a data bit pattern, or sets the start value of a pattern range.\n\nValid Values:\nBinary pattern string consisting of 1; 0; or X (any bit).\n\nAvailable Repeated Capabilities:\nNone\n\nRemote-control command(s):\nSEARch:TRIGger:DPHY:DATA:MIN"}, {"Level"=5, "Class Only"=FALSE, "Identifier"="RSSCOPE_ATTR_DPHY_SEARCH_HIGH_SPEED_DATA_MAX", "Descriptive Name"="DPHY Search High Speed Data Max", "Data Type"=2, "Command"="SEAR:TRIG:DPHY:DATA:MAX", "Access"=2, "Range Table"="", "Read Callback"="rsscope_FormatSearchNameString_ReadCallback.vi", "Write Callback"="rsscope_FormatSearchNameString_WriteCallback.vi", "Supported Models"="", "Instrument Options"="K42", "Flags"=0, "Help"="Sets the end value of a data type range for condition In Range or Out of Range. \n\nValid Values:\nBinary pattern string consisting of 1; 0; or X (any bit).\n\nAvailable Repeated Capabilities:\nNone\n\nRemote-control command(s):\nSEARch:TRIGger:DPHY:DATA:MAX"}, {"Level"=5, "Class Only"=FALSE, "Identifier"="RSSCOPE_ATTR_DPHY_SEARCH_LOW_POWER_ESCAPE_MODE_DATA_CONDITION", "Descriptive Name"="DPHY Search Low Power Escape Mode Data Condition", 
